vi "Decimate_Array.vi"() -> ()   [LabVIEW 2024]
panel:
  out "decimated array 2":dbl[](array[numeric])
  out "decimated array":dbl[](array[numeric])
  in  "array":dbl[](array[numeric])
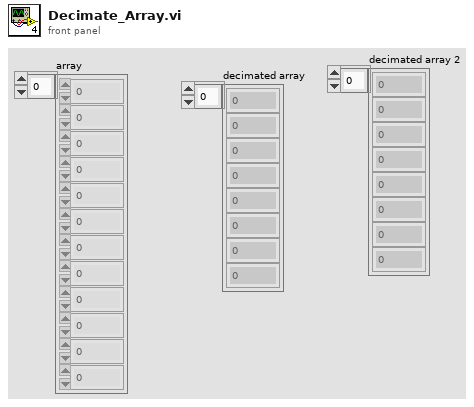
[diagram p1: front panel]
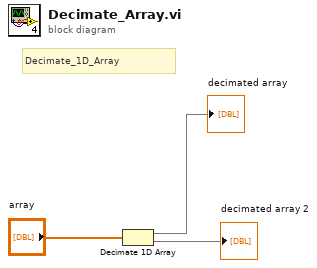
[diagram p0: block diagram]
diagram:
  # "Decimate_1D_Array"
  n1 = Decimate 1D Array("array") -> (→"decimated array":dbl[], →"decimated array 2":dbl[])
